vi "threshold-icator - i.vi"(6 "first time":bool=TRUE, 7 "requested size":i32=1, 10 "gamma":dbl, 11 "omega":dbl) -> (0 "last peak":dbl, 1 "new peak":bool, 2 "gamma array":dbl[](array[numeric]), 3 "omega array":dbl[](array[numeric]), 5 "array of peaks":dbl[](array[numeric]))   [LabVIEW 2015]
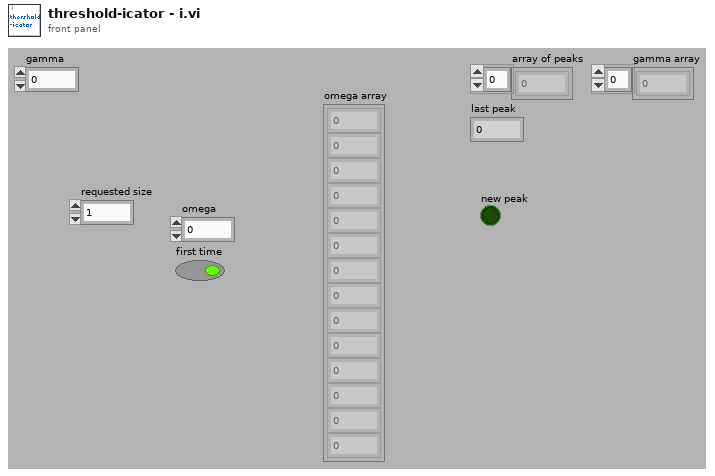
[diagram p1: front panel]
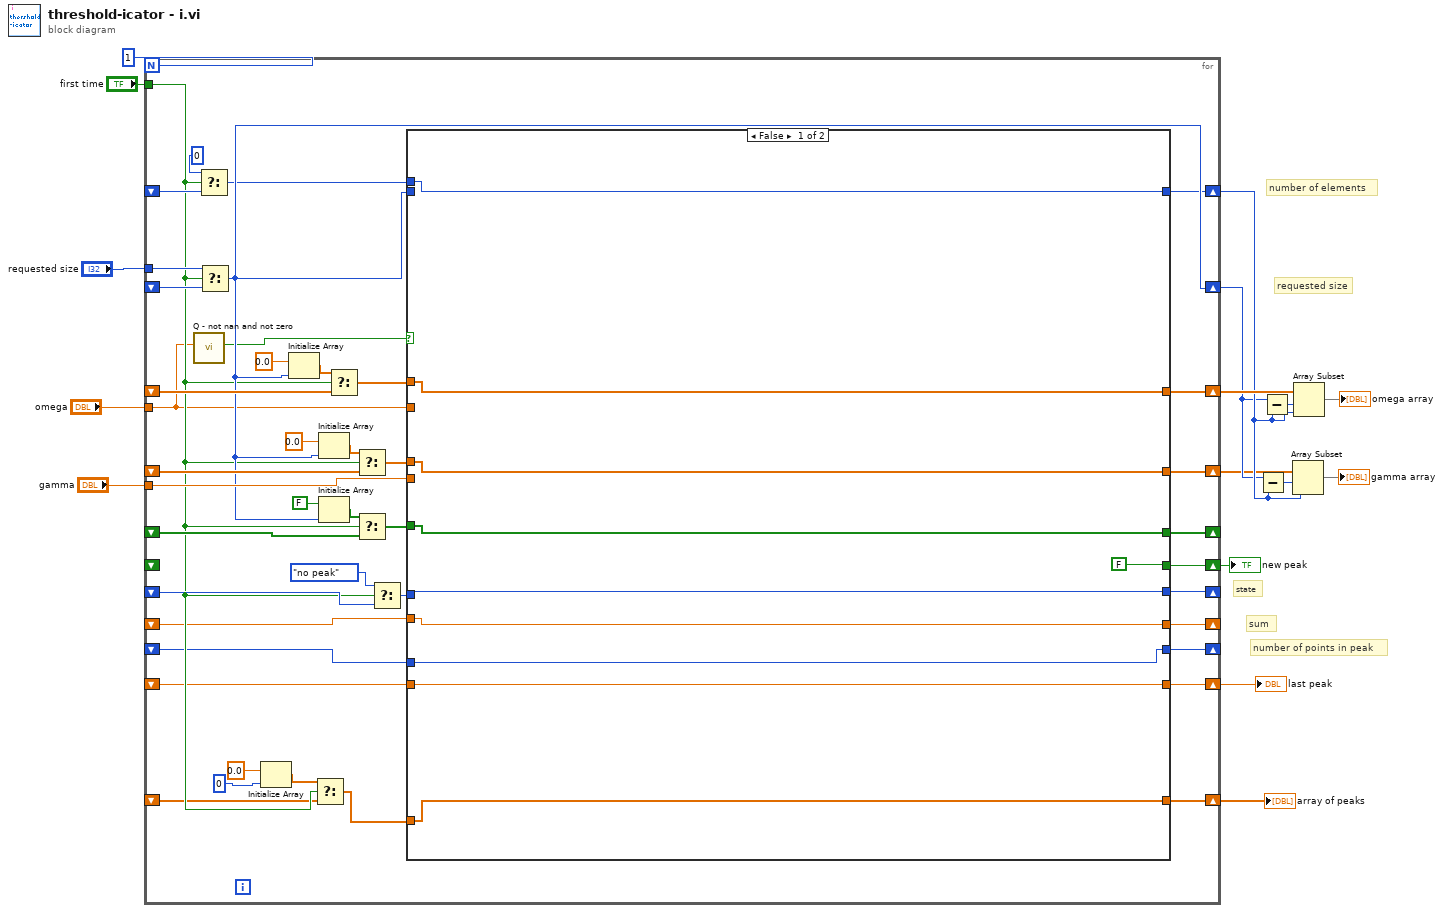
[diagram p0: block diagram]
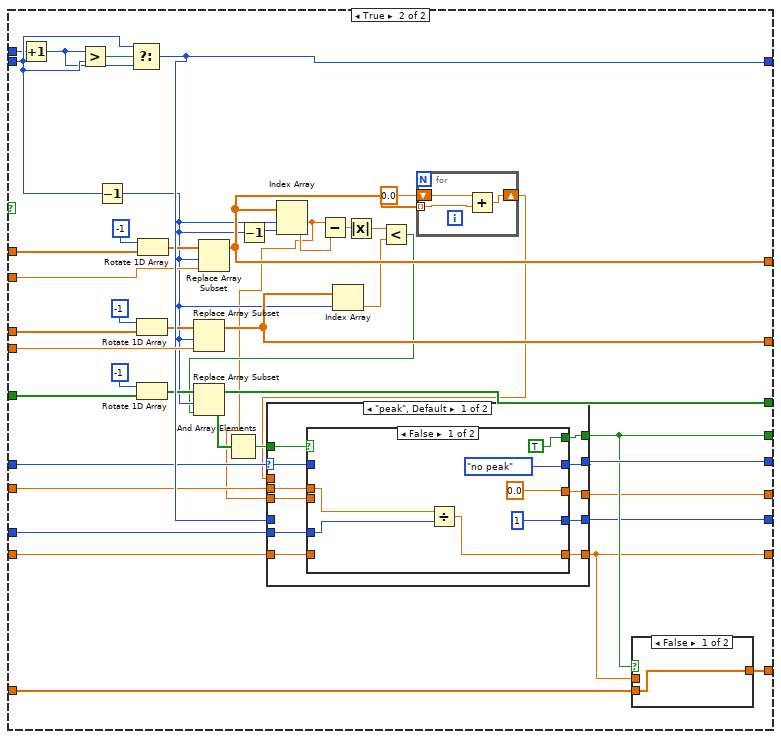
[diagram p2: hidden frame]
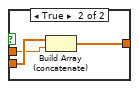
[diagram p3: hidden frame]
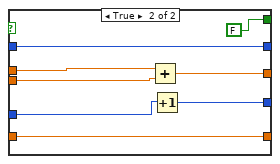
[diagram p4: hidden frame]
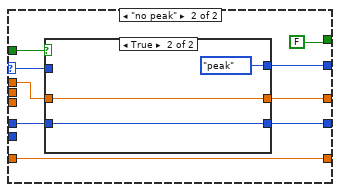
[diagram p5: hidden frame]
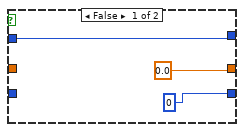
[diagram p6: hidden frame]
diagram:
  # "number of points in peak"
  # "sum"
  # "state"
  # "requested size"
  # "number of elements"
  n1 = for {
    N: 1 -> [_]
    tunnel: "first time" -> [w47]
    shift-right: [w41] -> w7
    shift-left: _ -> [w59]
    tunnel: "requested size" -> [w57]
    tunnel: "omega" -> [w35]
    shift-right: [w43] -> w12
    shift-left: _ -> [w58]
    shift-right: [w52] -> w6
    shift-left: _ -> [w56]
    shift-right: [w49] -> _
    shift-left: _ -> [w54]
    shift-right: [w50] -> w5
    shift-left: _ -> [w55]
    tunnel: "gamma" -> [w53]
    shift-right: [w44] -> _
    shift-left: _ -> [w51]
    shift-right: [w45] -> w1
    shift-left: _ -> [w46]
    shift-right: [w37] -> w2
    shift-left: _ -> [w36]
    shift-right: [w48] -> w3
    shift-left: _ -> [_]
    shift-right: [w42] -> _
    shift-left: _ -> [w39]
    shift-right: [w40] -> _
    shift-left: _ -> [w38]
    n2 = call "Q - not nan and not zero.vi"("Numeric"=w35) -> ("Boolean"=w17:bool)  [unwired: 10 in]
    n3 = Select(t=0, s=w47, f=w59) -> (s? t:f=w33:i32)
    n4 = Select(t=w57, s=w47, f=w56) -> (s? t:f=w52:i32)
    n5 = Initialize Array(0.0, 0) -> (w20:dbl[])
    n6 = Initialize Array(0.0, w52) -> (w31:dbl[])
    n7 = Select(t=w20, s=w47, f=w46) -> (s? t:f=w18:dbl[])
    n8 = Initialize Array(0.0, w52) -> (w28:dbl[])
    n9 = Initialize Array(FALSE, w52) -> (w24:bool[])
    n10 = Select(t=w31, s=w47, f=w58) -> (s? t:f=w30:dbl[])
    n11 = Select(t=w28, s=w47, f=w55) -> (s? t:f=w27:dbl[])
    n12 = Select(t=w24, s=w47, f=w51) -> (s? t:f=w23:bool[])
    n13 = Select(t=enum16{"peak", "no peak"}."no peak" ("Enum"), s=w47, f=w54) -> (s? t:f=w25:enum16{"peak", "no peak"})
    n14 = case shown="False" w17 {
      tunnel: w53 -> [_ w110]
      tunnel: w52 -> [_ w109]
      tunnel: [w67 w108] -> w50
      tunnel: [w64 w107] -> w49
      tunnel: [FALSE w106] -> w48
      tunnel: [w60 w105] -> w45
      tunnel: [w66 w104] -> w44
      tunnel: [w68 w103] -> w43
      tunnel: [w63 w102] -> w42
      tunnel: [w69 w101] -> w41
      tunnel: [w62 w100] -> w40
      tunnel: w39 -> [w63 w99]
      tunnel: w38 -> [w62 w98]
      tunnel: [w61 w97] -> w37
      tunnel: w36 -> [w61 w96]
      tunnel: w35 -> [_ w95]
      tunnel: w33 -> [w69 w93]
      tunnel: w30 -> [w68 w89]
      tunnel: w27 -> [w67 w88]
      tunnel: w25 -> [w64 w85]
      tunnel: w23 -> [w66 w84]
      tunnel: w18 -> [w60 w75]
      frame False {
      }
      frame True {
        n15 = Increment(x=w93) -> (x+1=w92:i32)
        n16 = Greater?(x=w92, y=w109) -> (0:w94:bool)
        n17 = Decrement(x=w109) -> (x-1=w78:i32)
        n18 = Select(t=w109, s=w94, f=w92) -> (s? t:f=w101:i32)
        n19 = Rotate 1D Array(1:w88, 2:-1 ("n")) -> (0:w86:dbl[])
        n20 = Rotate 1D Array(1:w84, 2:-1 ("n")) -> (0:w82:bool[])
        n21 = Rotate 1D Array(1:w89, 2:-1 ("n")) -> (0:w90:dbl[])
        n22 = Replace Array Subset(array=w86, new element=w110, index=w78) -> (w108:dbl[])
        n23 = Replace Array Subset(array=w90, new element=w95, index=w78) -> (w103:dbl[])
        n24 = Decrement(x=w78) -> (x-1=w81:i32)
        n25 = Index Array(array=w103, index #1=w78, index #2=w81) -> (element #1=w70:dbl, element #2=w74:dbl)
        n26 = Subtract(x=w70, y=w74) -> (x-y=w80:dbl)
        n27 = Index Array(array=w108, index=w78) -> (element=w77:dbl)
        n28 = Absolute Value(x=w80) -> (abs(x)=w79:dbl)
        n29 = Less?(x=w79, y=w77) -> (x < y?=w76:bool)
        n30 = Replace Array Subset(array=w82, new element=w76, index=w78) -> (w104:bool[])
        n31 = And Array Elements(Boolean array=w104) -> (logical AND=w73:bool)
        n32 = for {
          tunnel: w103 -> [w112] mode=indexing
          shift-right: [w111] -> w71
          shift-left: 0.0 -> [w113]
          n33 = Add(x=w113, y=w112) -> (x+y=w111:dbl)
        }
        n34 = case shown="\"peak\", Default" w85 {
          selector: w85 -> [w127 w151]
          tunnel: [w128 w152] -> w107
          tunnel: [w126 FALSE] -> w106
          tunnel: w73 -> [w125 w149]
          tunnel: w71 -> [_ w148]
          tunnel: [w122 w147] -> w102
          tunnel: w101 -> [_ w146]
          tunnel: [w120 w145] -> w100
          tunnel: w70 -> [w124 _]
          tunnel: w99 -> [w123 _]
          tunnel: w98 -> [w121 _]
          tunnel: [w119 w144] -> w97
          tunnel: w96 -> [w118 w144]
          frame "peak", Default {
            n35 = case shown="False" w125 {
              tunnel: [enum16{"peak", "no peak"}."no peak" ("Enum") w143] -> w128
              tunnel: w127 -> [_ w143]
              tunnel: [TRUE FALSE] -> w126
              tunnel: w124 -> [_ w141]
              tunnel: w123 -> [w133 w140]
              tunnel: [0.0 w139] -> w122
              tunnel: w121 -> [w132 w138]
              tunnel: [1 w137] -> w120
              tunnel: [w131 w136] -> w119
              tunnel: w118 -> [_ w136]
              frame False {
                n36 = Divide(x=w133, y=w132) -> (x/y=w131:dbl)
              }
              frame True {
                n37 = Add(x=w140, y=w141) -> (x+y=w139:dbl)
                n38 = Increment(x=w138) -> (x+1=w137:i32)
              }
            }
          }
          frame "no peak" {
            n39 = case shown="True" w149 {
              tunnel: [w155 enum16{"peak", "no peak"}."peak" ("Enum")] -> w152
              tunnel: w151 -> [w155 _]
              tunnel: w148 -> [_ w157]
              tunnel: [0.0 w157] -> w147
              tunnel: w146 -> [_ w156]
              tunnel: [0 w156] -> w145
              frame False {
              }
              frame True {
              }
            }
          }
        }
        n40 = case shown="False" w106 {
          tunnel: w75 -> [w114 w117]
          tunnel: w97 -> [_ w116]
          tunnel: [w114 w115] -> w105
          frame False {
          }
          frame True {
            n41 = Build Array (concatenate)(w117, w116) -> (w115:dbl[])
          }
        }
      }
    }
  }
  "array of peaks" <- w1
  "last peak" <- w2
  "new peak" <- w3
  n42 = Subtract(x=w6, y=w7) -> (x-y=w9:i32)
  n43 = Subtract(x=w6, y=w7) -> (x-y=w10:i32)
  n44 = Array Subset(array=w5, index=w9, length=w7) -> (→"gamma array":dbl[])
  n45 = Array Subset(array=w12, index=w10, length=w7) -> (→"omega array":dbl[])
